vi "initialize nested actor.vi"(8 "error in (no error)":errorcluster, 11 "Template in":refnum<class "Template.lvclass">) -> (0 "error out":errorcluster, 3 "Template out":refnum<class "Template.lvclass">)   [LabVIEW 2020, in "Template.lvlib" / "Template.lvclass"]
uses:
  Template.lvclass
  Template.lvclass/Template.ctl
  accessors/Read This Actor Number.vi
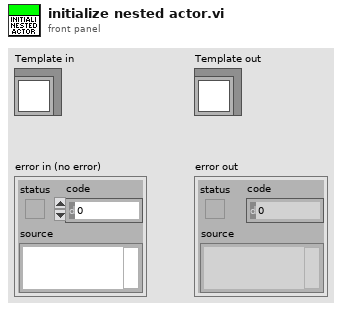
[diagram p1: front panel]
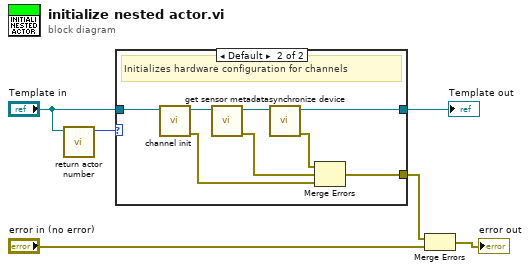
[diagram p0: block diagram]
diagram:
  n1 = call "return actor number.vi"("Template in"="Template in") -> ("Actor number"=w1:u32)  [unwired: 10 in]
  n2 = case shown="Default" w1 {
    tunnel: [_ w13] -> w4
    tunnel: "Template in" -> [w7 w12]
    tunnel: [w7 w10] -> w2
    frame 0 {
      # "Actor 0 has no hardware interface. Do nothing here."
    }
    frame Default {
      # "Initializes hardware configuration for channels"
      n3 = call-dynamic "channel init.vi"("Template in"=w12) -> ("error out"=w8:errorcluster, "Template out"=w9:refnum<class "Template.lvclass">)  [unwired: 9 in]
      n4 = call-dynamic "get sensor metadata.vi"("Template in"=w9) -> ("error out"=w14:errorcluster, "Template out"=w11:refnum<class "Template.lvclass">)  [unwired: 9 in]
      n5 = call-dynamic "synchronize device.vi"("Template in"=w11) -> ("error out"=w15:errorcluster, "Template out"=w10:refnum<class "Template.lvclass">)  [unwired: 9 in]
      n6 = Merge Errors(w15, w14, w8) -> (w13:errorcluster)
    }
  }
  "Template out" <- w2
  n7 = Merge Errors(w4, "error in (no error)") -> (→"error out":errorcluster)
